vi "Get Request Type.vi"(8 "error in (no error)":errorcluster, 11 "SetCurrentProfile in":refnum<class "SetCurrentProfile.lvclass">) -> (0 "error out":errorcluster, 2 "Request Type":string, 3 "SetCurrentProfile out":refnum<class "SetCurrentProfile.lvclass">)   [LabVIEW 2020, in "obs-websocket.lvlib" / "SetCurrentProfile.lvclass"]
uses:
  SetCurrentProfile.lvclass
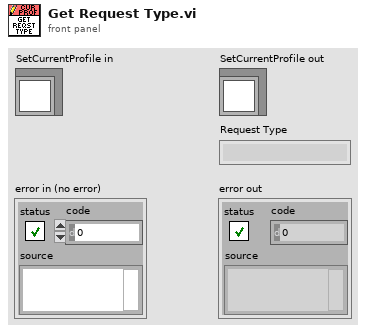
[diagram p1: front panel]
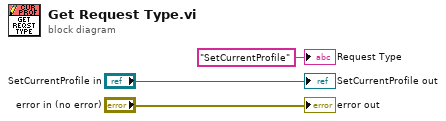
[diagram p0: block diagram]
diagram:
  "error out" <- "error in (no error)"
  "SetCurrentProfile out" <- "SetCurrentProfile in"
  "Request Type" <- "SetCurrentProfile" ("Request Type")
